vi "Move Down UP.vi"(8 "Distance Up":dbl, 11 "Distance Down":dbl) -> ()   [LabVIEW 2014]
uses:
  Global Variables.vi
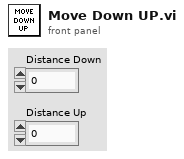
[diagram p1: front panel]
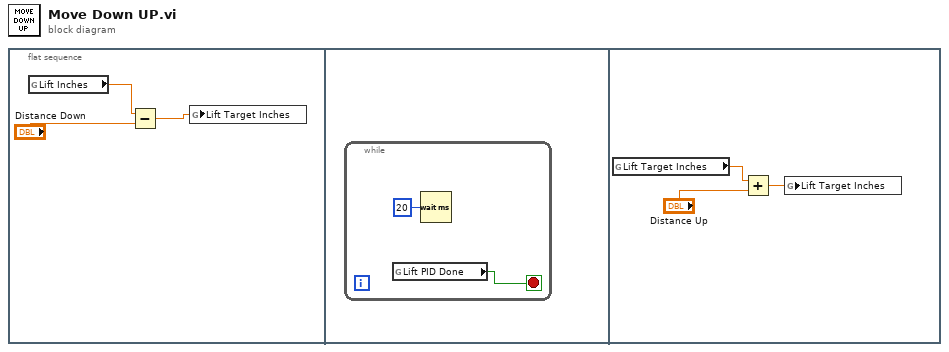
[diagram p0: block diagram]
diagram:
  n1 = flat-sequence {
    frame #0 {
      n2 = global read "Global Variables.vi" "Lift Inches"() -> (w3:dbl)
      n3 = Subtract(x=w3, y="Distance Down") -> (x-y=w1:dbl)
      n4 = global write "Global Variables.vi" "Lift Target Inches"(w1) -> ()
    }
    frame #1 {
      n5 = while {
        stop <- w5 stop-if-true
        n6 = global read "Global Variables.vi" "Lift PID Done"() -> (w5:bool)
        n7 = Wait (ms)(milliseconds to wait=u32 20) -> ()  [unwired: 1 out]
      }
    }
    frame #2 {
      n8 = global read "Global Variables.vi" "Lift Target Inches"() -> (w7:dbl)
      n9 = Add(x=w7, y="Distance Up") -> (x+y=w6:dbl)
      n10 = global write "Global Variables.vi" "Lift Target Inches"(w6) -> ()
    }
  }
